vi "tm_getframe8_40.vi"(7 "Options":i32(ring) items=["no option"=0, "high contrast"=16], 8 "error in (no error)":errorcluster {"code" format="%.0x"}, 10 "Frame Index":i32=-1, 11 "Handle in":u32) -> (0 "error out":errorcluster {"code" format="%.0x"}, 1 "Timestamp":dbl, 2 "Data":u8[][](array[numeric]), 3 "Handle out":u32)   [LabVIEW 2023]
uses:
  tmcamcon.dll
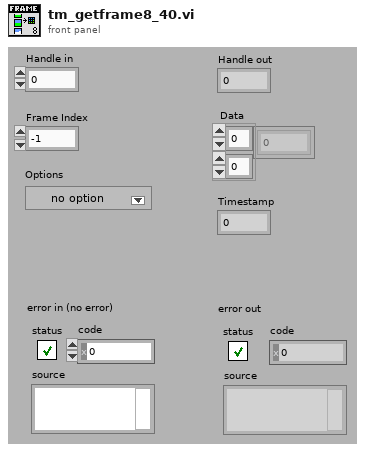
[diagram p1: front panel]
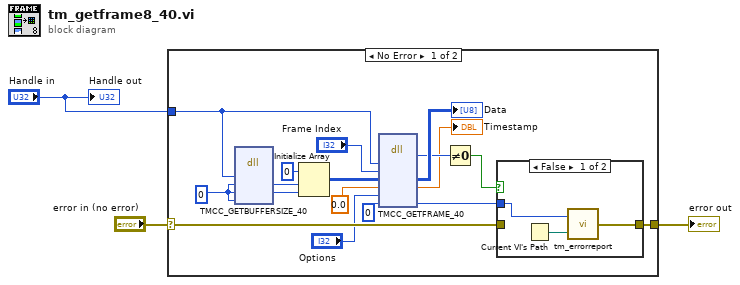
[diagram p0: block diagram]
diagram:
  n1 = case shown="No Error" "error in (no error)" {
    selector: "error in (no error)" -> [w18 w25]
    tunnel: [w17 w25] -> w2
    tunnel: "Handle in" -> [w10 _]
    frame No Error {
      w7 = 0 ("width")
      n2 = dll-call lib="tmcamcon.dll" fn="TMCC_GETBUFFERSIZE_40"("index"=w10, "height"=w7, "width"=w7, "Erval"=w7) -> ("height"=w9:i32, "width"=w8:i32)  [unwired: 6 in, 2 out]
      n3 = Initialize Array(u8 0, w9, w8) -> (w12:u8[][])
      n4 = dll-call lib="tmcamcon.dll" fn="TMCC_GETFRAME_40"("index"=w10, "frameindex"="Frame Index", "imgarray"=w12, "timestamp"=0.0, "option"="Options", "Erval"=0) -> ("return type"=w11:u32, "imgarray"=→"Data":u8[][], "timestamp"=→"Timestamp":dbl, "Erval"=w16:i32)  [unwired: 6 in, 2 out]
      n5 = Not Equal To 0?(x=w11) -> (x != 0?=w15:bool)
      n6 = case shown="False" w15 {
        tunnel: w18 -> [_ w24]
        tunnel: [w22 w24] -> w17
        tunnel: w16 -> [w21 _]
        frame False {
          n7 = Current VI's Path() -> (path=w23:path)
          n8 = call "tm_errorreport.vi"("Source"=w23, "Error"=w21) -> ("error out"=w22:errorcluster)
        }
        frame True {
        }
      }
    }
    frame Error {
    }
  }
  "error out" <- w2
  "Handle out" <- "Handle in"
